vi "Dual_image_synced_p_read.vi"() -> ()   [LabVIEW 2013]
uses:
  <vilib>/DAQmx/write.llb/DAQmx Write (Analog DBL 1Chan 1Samp).vi
  <vilib>/DAQmx/create/channels.llb/DAQmx Create Channel (AO-Voltage-Basic).vi
  <vilib>/DAQmx/create/channels.llb/DAQmx Create Channel (CO-Pulse Generation-Frequency).vi
  <vilib>/DAQmx/configure/timing.llb/DAQmx Timing (Implicit).vi
  <vilib>/DAQmx/miscellaneous.llb/DAQmx Fill In Error Info.vi
  <vilib>/vision/driver/NI_Vision_Acquisition_Software.lvlib
  <resource>/objmgr/imaqdx.rc
  <resource>/objmgr/daqmx.rc
panel:
  in  "Pressure Frequency (Hz)":dbl=10.0 format="%#_13g"
  in  "im num 2":string
  in  "im time 2":string
  out "im num":string
  out "im time":string
  out "Pressure Reading":cluster{dbl[], dbl[]}(graph)
  in  "Pressure Offset":dbl
  out "Current Pressure (Psi)":dbl format="%#.4g"
  in  "Gain 2":dbl(slide)=575.0 min=350.0 max=1000.0 step=1.0 scale=350.0..1000.0
  in  "VR2":dbl(slide)=65.0 min=0.0 max=255.0 step=1.0 scale=0.0..255.0
  in  "VR1":dbl(slide)=60.0 min=0.0 max=255.0 step=1.0 scale=0.0..255.0
  in  "UB2":dbl(slide)=160.0 min=0.0 max=255.0 step=1.0 scale=0.0..255.0
  in  "UB1":dbl(slide)=165.0 min=0.0 max=255.0 step=1.0 scale=0.0..255.0
  in  "Shutter":dbl(slide)=4095.0 min=0.0 max=4095.0 step=1.0 scale=4.095..4095.0 scale format="%#.0f"
  in  "Brightness":dbl(slide)=100.0 min=0.0 max=255.0 step=1.0 scale=0.0..255.0
  in  "Gain":dbl(slide)=600.0 min=350.0 max=1000.0 step=1.0 scale=350.0..1000.0
  in  "Test Description":string="test"
  in  "Storage Directory":path=path "C:/Users/Regen/Desktop/Users/Ryan Gergely/3D_DIC"
  out "Image 2":T1(plugin-control)
  out "Buffer Number 2":u32
  out "Frame Rate 2":dbl
  in  "Camera Name 2":refnum<k21>="cam2" caption="IMAQdx Session"
  in  "Image Frequency (Hz)":dbl=2.0 format="%.1f"
  out "Actual Duty Cycle":dbl
  out "Actual Frequency":dbl
  in  "Stop":bool
  in  "Start Trigger Mode":bool
  out "Frame Rate 1":dbl
  out "Buffer Number 1":u32
  in  "Camera Name 1":refnum<k21>="cam1" caption="IMAQdx Session"
  out "Image":T1(plugin-control)
  # "Exposure Settings - Both Cameras"
  # "White Balance - Camera1"
  # "White Balance - Camera2"
  # "1) Set Test Description and Storage Directory"
  # "2) Select Cameras"
  # "3) Start VI"
  # "4) Set Frequency and Exposure and White Balance\n(Before Start Trigger)"
  # "5)"
  # "6) Stop When Done"
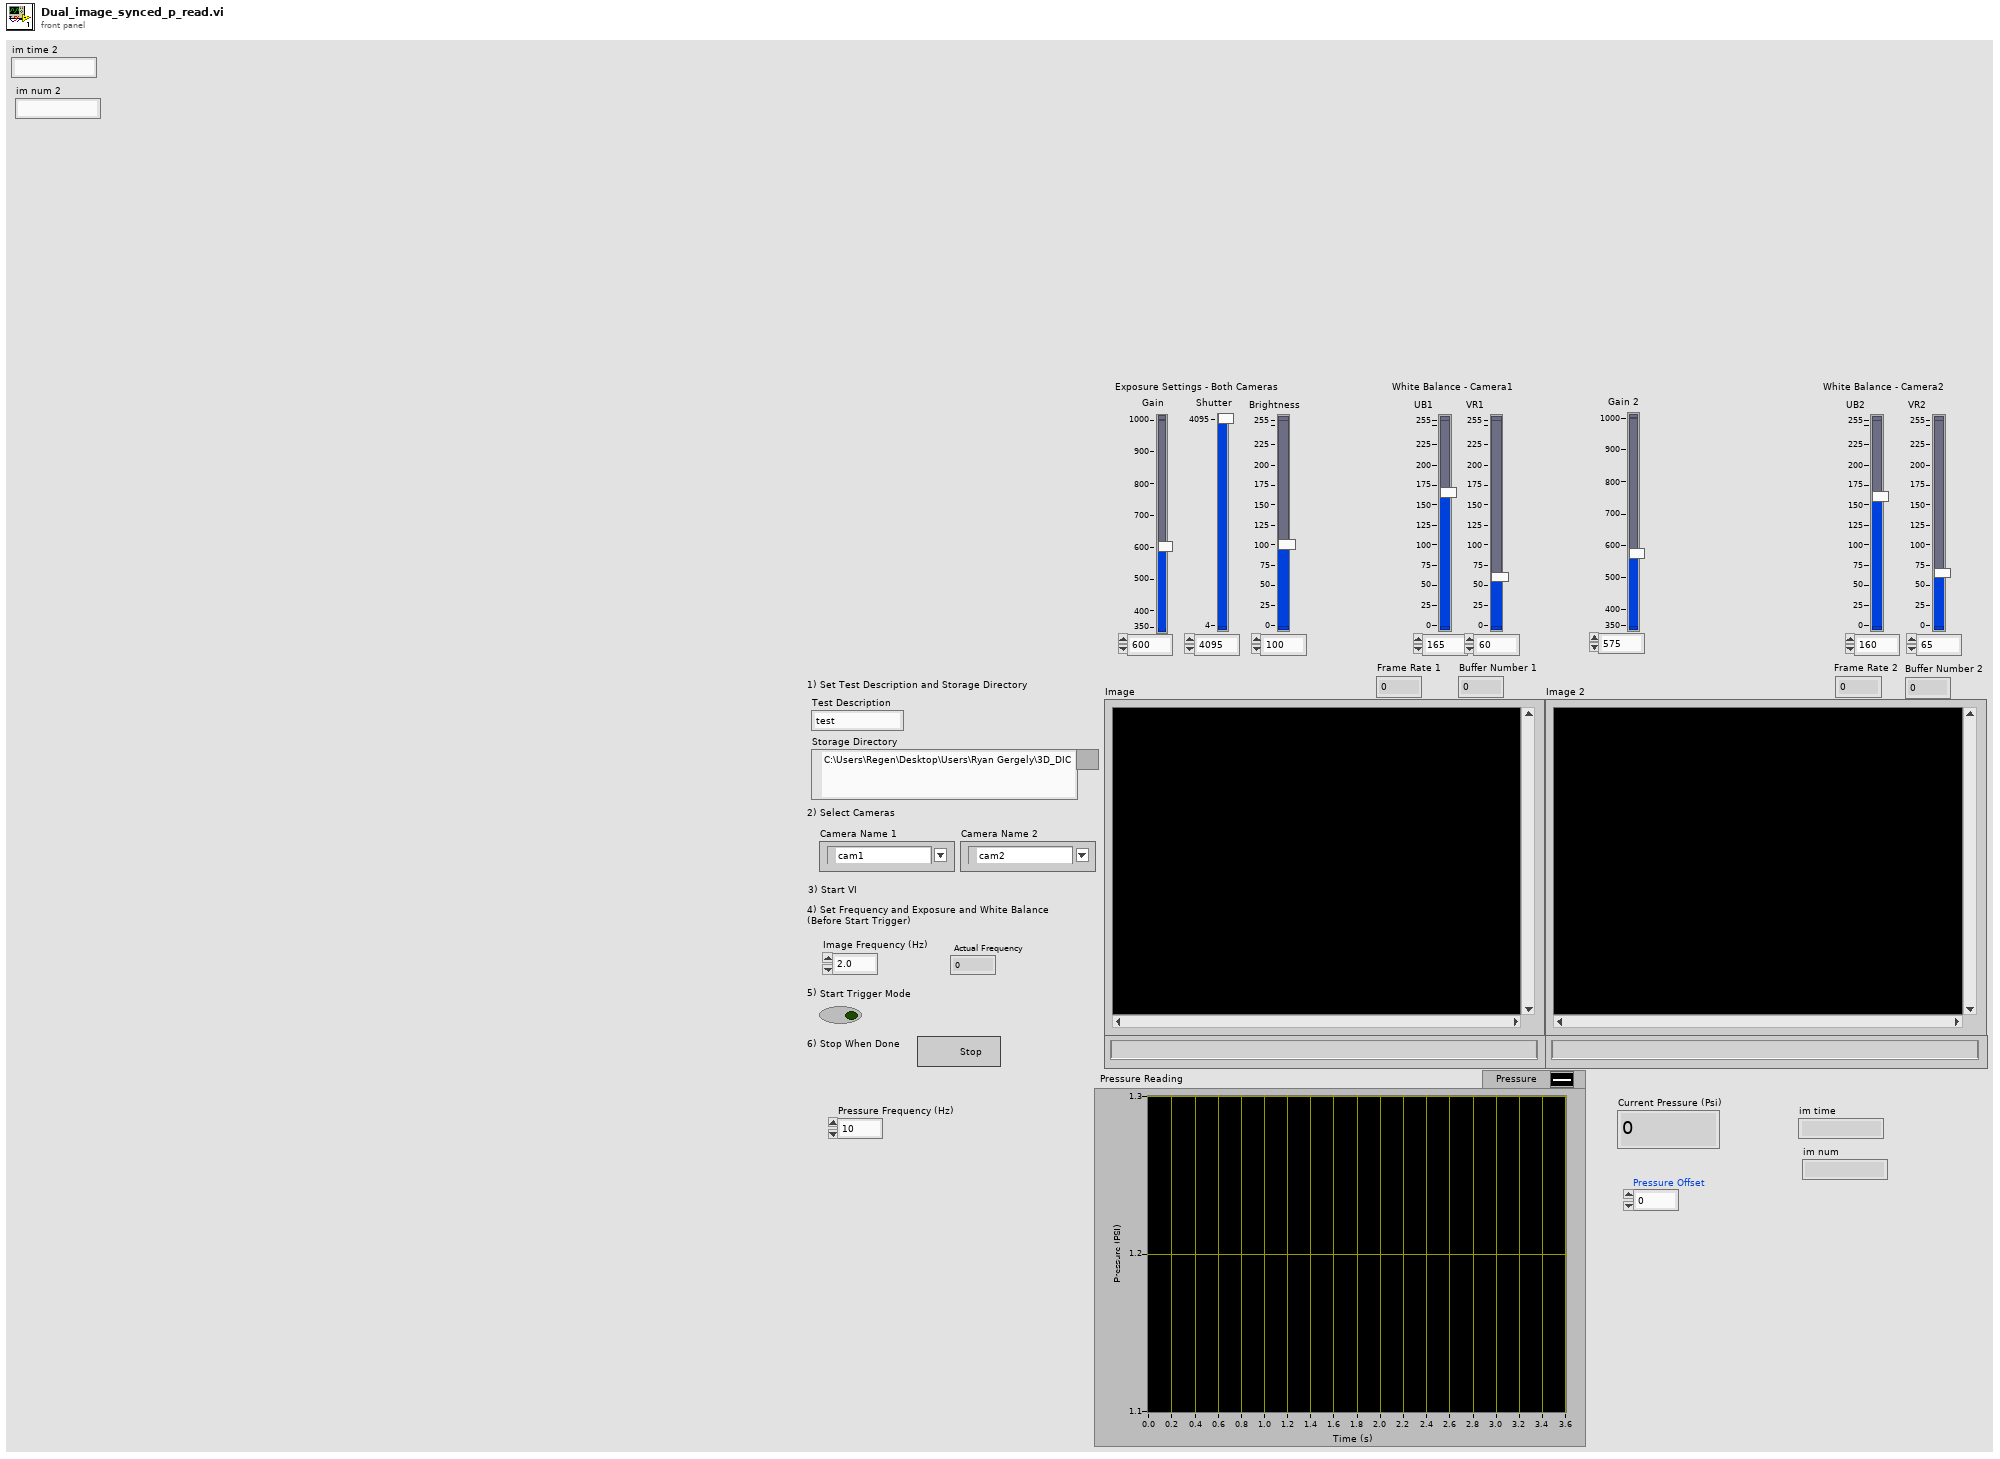
[diagram p1: front panel]
types:
  T1 = typedef "IMAQ Image.ctl" = refnum<image>
  T2 = enum16{"open", "open or create", "create or replace", "create", "open (read only)"}
  T3 = typedef "IMAQdx.ctl" = refnum<k21>
  T4 = cluster{"Trigger Mode":u32, "Trigger Activation":u32, "Timeout (ms)":u32}
  T5 = enum16{"open", "replace", "create", "open or create", "replace or create", "replace or create with confirmation"}
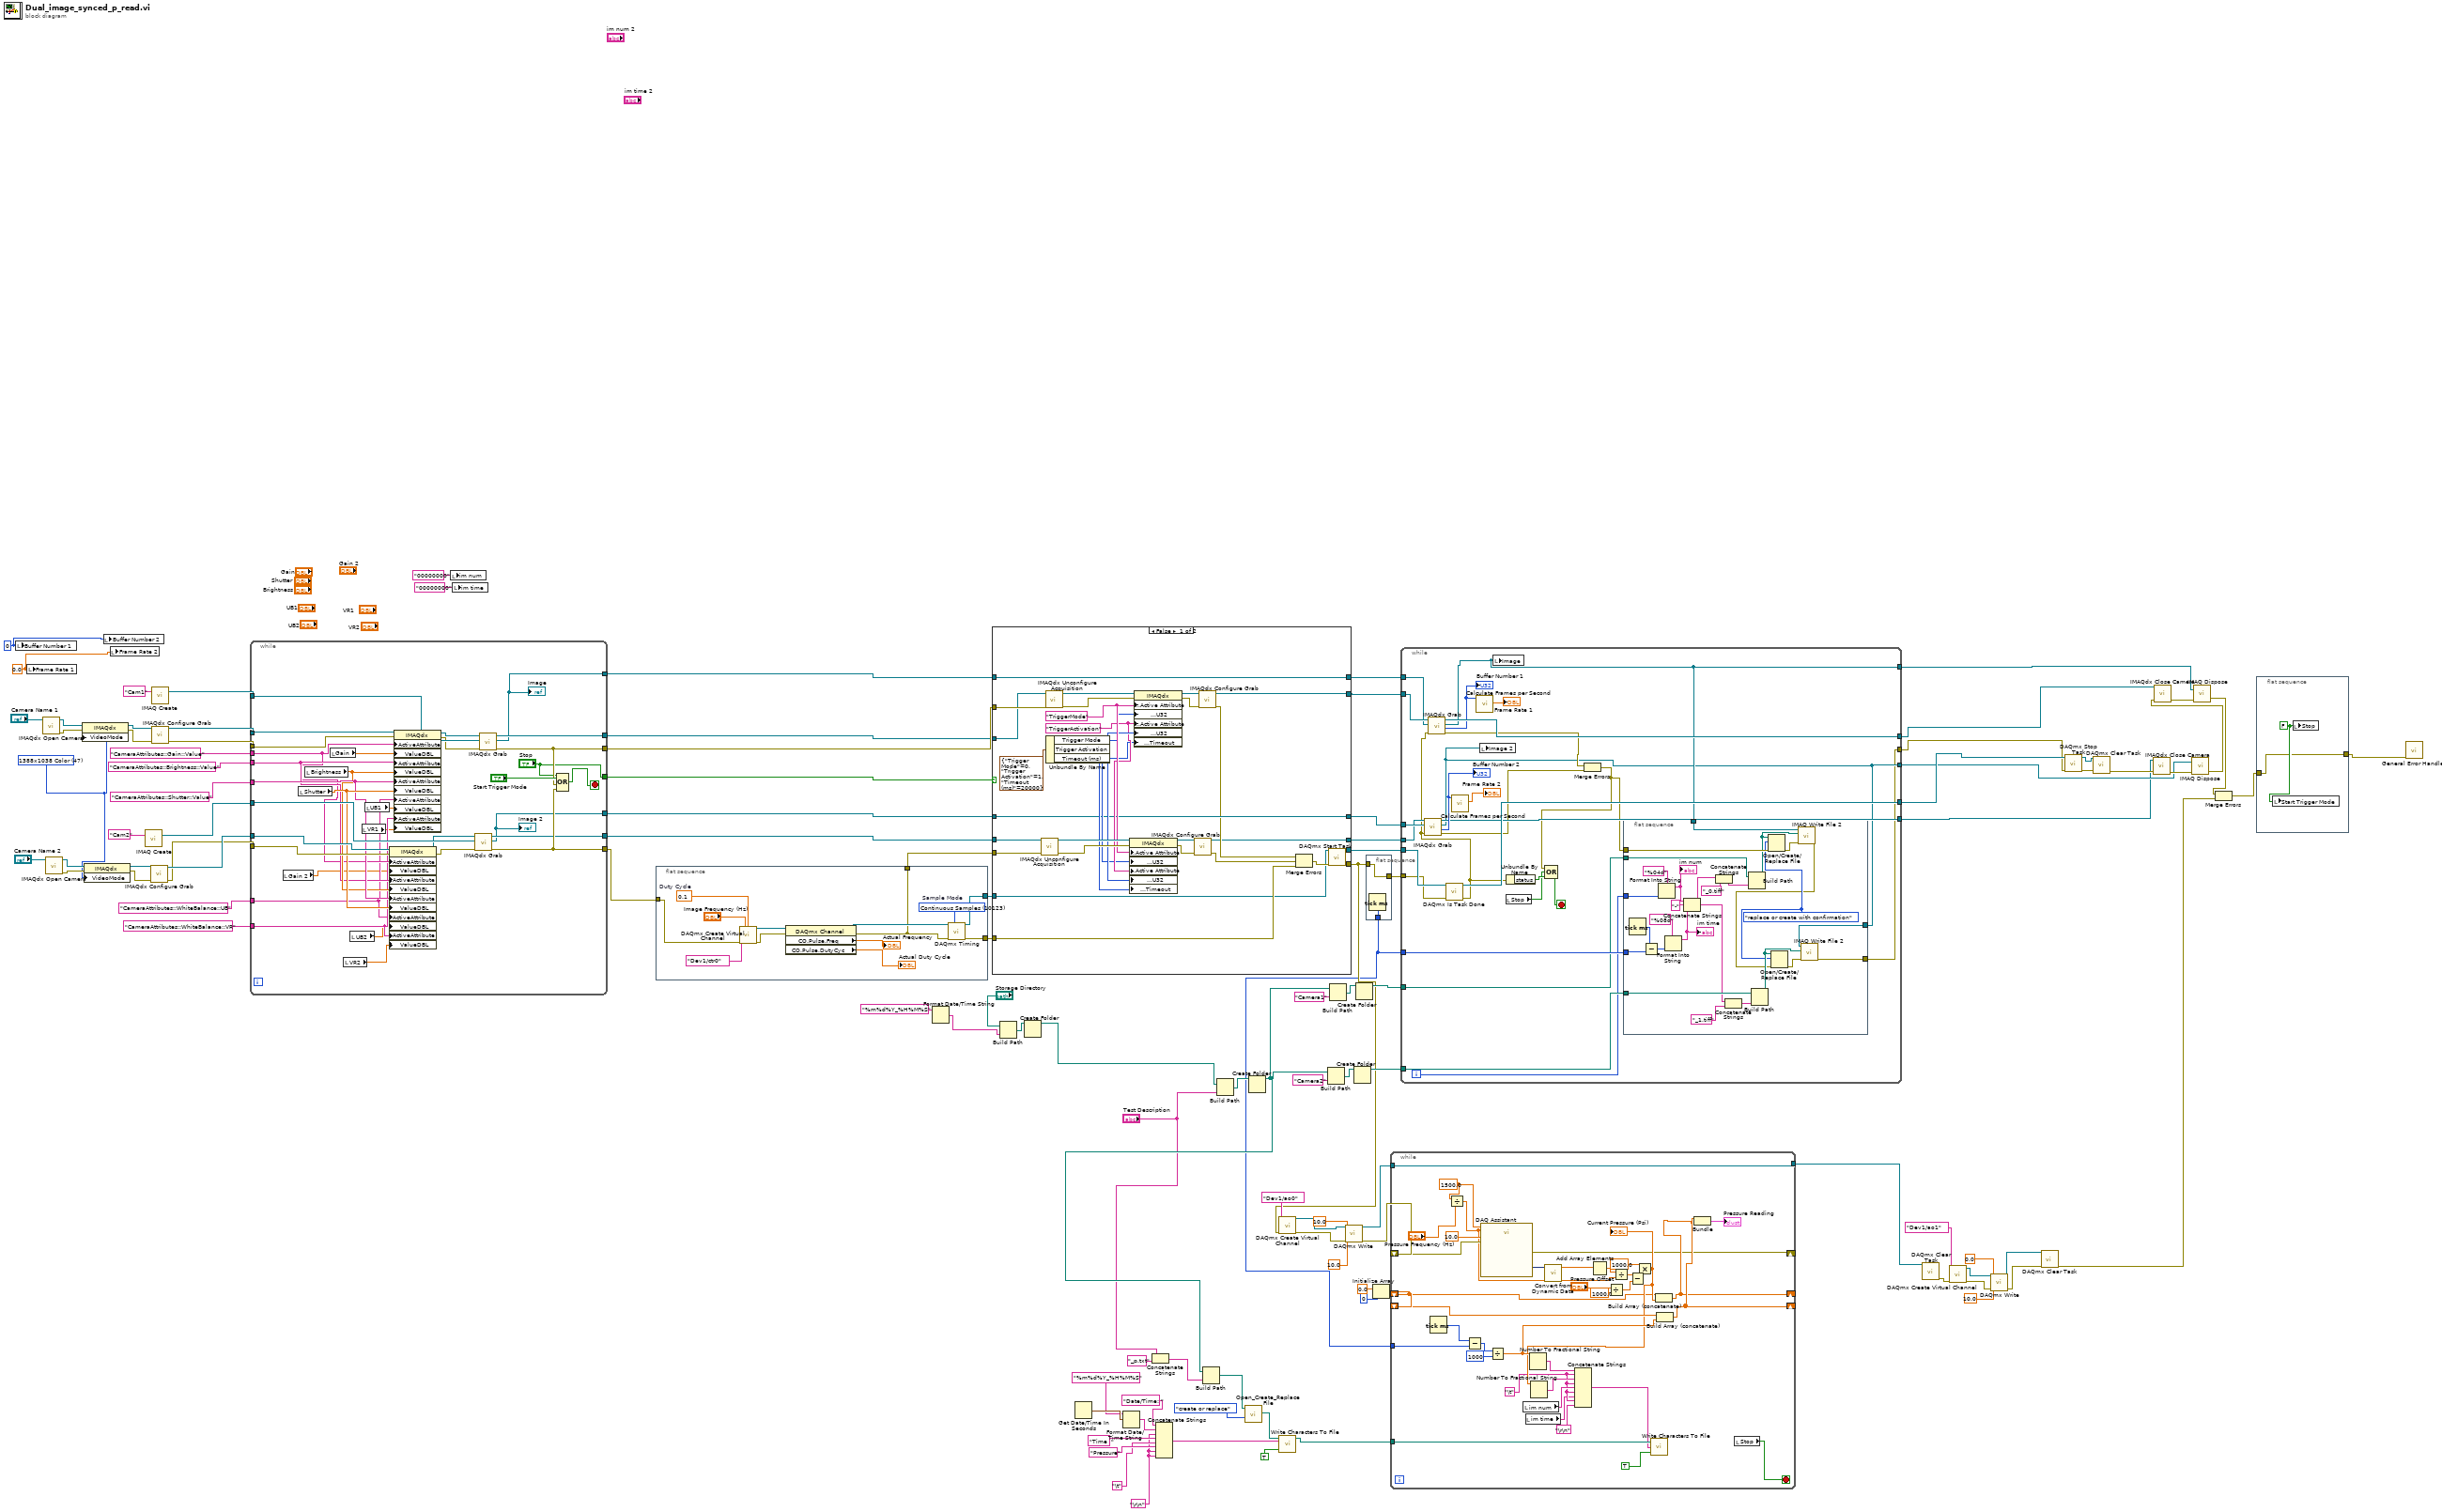
[diagram p0: block diagram]
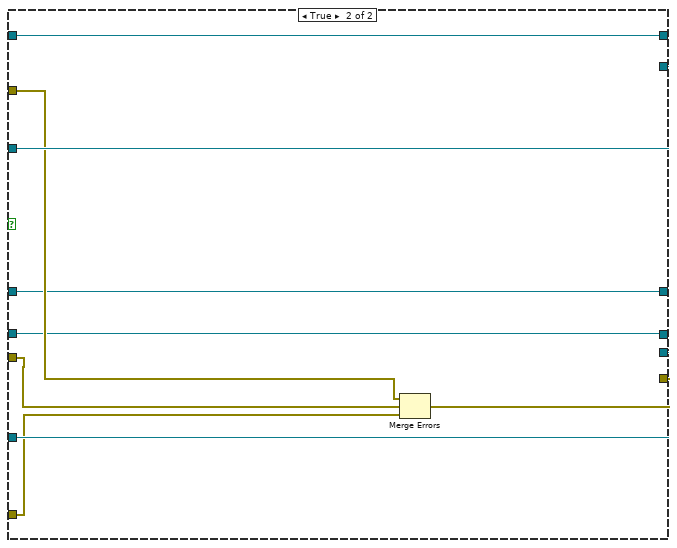
[diagram p2: hidden frame]
diagram:
  w34 = "\r\n"
  w57 = u32 47 items=["320x240 Color"=4, "640x480 Mono8"=9, "640x480 Mono16"=19, "640x480 Color"=14, "800x600 Mono8"=21, "800x600 Mono16"=27, "800x600 Color"=24, "1024x768 Mono8"=30, "1024x768 Mono16"=36, "1024x768 Color"=33, "1280x960 Mono8"=40, "1280x960 Mono16"=46, "1280x960 Color"=43, "1388x1038 Color"=47, "1388x1038 Mono"=48] ("Video Mode")
  w58 = 0.0 ("Frame Rate 1")
  w59 = u32 0 ("Buffer Number 1")
  n1 = local write "Buffer Number 1"(w59) -> ()
  n2 = local write "Frame Rate 1"(w58) -> ()
  n3 = call <vilib>:"IMAQdx Open Camera.vi"("Session In"="Camera Name 1") -> ("error out"=w65:errorcluster, "Session Out"=w67:T3)  [unwired: 2 in, 7 out]
  n4 = call <vilib>:"IMAQdx Open Camera.vi"("Session In"="Camera Name 2") -> ("error out"=w60:errorcluster, "Session Out"=w61:T3)  [unwired: 2 in, 7 out]
  n5 = property class="IMAQdx"(reference=w67, error in=w65, "VideoMode"=w57) -> (reference out=w66:T3, error out=w64:errorcluster)
  n6 = property class="IMAQdx"(reference=w61, error in=w60, "VideoMode"=w57) -> (reference out=w63:T3, error out=w62:errorcluster)
  n7 = local write "Buffer Number 2"(w59) -> ()
  n8 = local write "Frame Rate 2"(w58) -> ()
  n9 = call "IMAQ Create"("Image Name"="Cam2") -> ("New Image"=w54:T1)  [unwired: 3 in, 2 out]
  n10 = call <vilib>:"IMAQdx Configure Grab.vi"("error in"=w62, "Session In"=w63) -> ("error out"=w90:errorcluster, "Session Out"=w91:T3)  [unwired: 8 out]
  n11 = call "IMAQ Create"("Image Name"="Cam1") -> ("New Image"=w101:T1)  [unwired: 3 in, 2 out]
  n12 = call <vilib>:"IMAQdx Configure Grab.vi"("error in"=w64, "Session In"=w66) -> ("error out"=w99:errorcluster, "Session Out"=w100:T3)  [unwired: 8 out]
  n13 = while {
    tunnel: [w143] -> w108
    tunnel: w99 -> [w130]
    tunnel: w100 -> [w132]
    tunnel: [w139] -> w109
    tunnel: w101 -> [w134]
    tunnel: [w142] -> w96
    tunnel: ["Stop"] -> w97
    tunnel: w91 -> [w128]
    tunnel: w90 -> [w127]
    tunnel: [w137] -> w56
    tunnel: [w136] -> w89
    tunnel: [w135] -> w88
    tunnel: w54 -> [w133]
    tunnel: "CameraAttributes::Shutter::Value" ("ActiveAttribute") -> [w123]
    tunnel: "CameraAttributes::Brightness::Value" ("ActiveAttribute") -> [w121]
    tunnel: "CameraAttributes::Gain::Value" ("ActiveAttribute") -> [w119]
    tunnel: "CameraAttributes::WhiteBalance::UB" ("ActiveAttribute") -> [w116]
    tunnel: "CameraAttributes::WhiteBalance::VR" ("ActiveAttribute") -> [w117]
    stop <- w140 stop-if-true
    n14 = local read "Gain 2"() -> (w112:dbl)
    n15 = local read "Shutter"() -> (w124:dbl)
    n16 = local read "Brightness"() -> (w122:dbl)
    n17 = local read "Gain"() -> (w120:dbl)
    n18 = local read "VR2"() -> (w113:dbl)
    n19 = local read "UB2"() -> (w115:dbl)
    n20 = local read "VR1"() -> (w114:dbl)
    n21 = local read "UB1"() -> (w118:dbl)
    n22 = property class="IMAQdx"(reference=w128, error in=w127, "ActiveAttribute"=w119, "ValueDBL"=w112, "ActiveAttribute"=w121, "ValueDBL"=w122, "ActiveAttribute"=w123, "ValueDBL"=w124, "ActiveAttribute"=w116, "ValueDBL"=w115, "ActiveAttribute"=w117, "ValueDBL"=w113) -> (reference out=w125:T3, error out=w126:errorcluster)
    n23 = property class="IMAQdx"(reference=w132, error in=w130, "ActiveAttribute"=w119, "ValueDBL"=w120, "ActiveAttribute"=w121, "ValueDBL"=w122, "ActiveAttribute"=w123, "ValueDBL"=w124, "ActiveAttribute"=w116, "ValueDBL"=w118, "ActiveAttribute"=w117, "ValueDBL"=w114) -> (reference out=w131:T3, error out=w129:errorcluster)
    n24 = call <vilib>:"IMAQdx Grab.vi"("error in"=w126, "Image In"=w133, "Session In"=w125) -> ("error out"=w137:errorcluster, "Image Out"=w135:T1, "Session Out"=w136:T3)  [unwired: 1 in, 5 out]
    "Image 2" <- w135
    n25 = call <vilib>:"IMAQdx Grab.vi"("error in"=w129, "Image In"=w134, "Session In"=w131) -> ("error out"=w139:errorcluster, "Image Out"=w142:T1, "Session Out"=w143:T3)  [unwired: 1 in, 5 out]
    "Image" <- w142
    n26 = Compound Arithmetic op=OR("Stop", "Start Trigger Mode", w139, w137) -> (w140:bool)
  }
  n27 = local write "im num"("00000000" ("im num 2")) -> ()
  n28 = local write "im time"("00000000" ("im time 2")) -> ()
  n29 = flat-sequence {
    tunnel: [w147] -> w94
    tunnel: [w146] -> w87
    tunnel: w56 -> [w145]
    tunnel: [w144] -> w55
    frame #0 {
      w154 = 0.1  # Duty Cycle
      w148 = 10123 items=["Finite Samples"=10178, "Continuous Samples"=10123, "Hardware Timed Single Point"=12522]  # Sample Mode
      n30 = call-poly <vilib>:"DAQmx Create Virtual Channel.vi"("frequency"="Image Frequency (Hz)", "duty cycle"=w154, "counter"=tag "Dev1/ctr0" ("Counter"), "error in"=w145) -> ("task out"=w150:refnum<k21>, "error out"=w151:errorcluster)  [unwired: 10 in]
      n31 = property class="DAQmx Channel"(reference=w150, error in=w151) -> (reference out=w152:refnum<k21>, error out=w144:errorcluster, "CO.Pulse.Freq"=→"Actual Frequency":dbl, "CO.Pulse.DutyCyc"=→"Actual Duty Cycle":dbl)
      n32 = call-poly <vilib>:"DAQmx Timing.vi"("task/channels in"=w152, "sample mode"=w148, "error in"=w144) -> ("task out"=w147:refnum<k21>, "error out"=w146:errorcluster)  [unwired: 11 in]
    }
  }
  n33 = Format Date/Time String(time format string (%c)="%m%d%Y_%H%M%S") -> (date/time string=w76:string)  [unwired: 2 in]
  n34 = case shown="False" w97 {
    tunnel: w109 -> [w185 w191]
    tunnel: w108 -> [w184 w194]
    tunnel: [w183 w194] -> w107
    tunnel: [w164 w190] -> w9
    tunnel: [w165 w192] -> w105
    tunnel: w96 -> [w177 w193]
    tunnel: [w177 w193] -> w95
    tunnel: w94 -> [w157 w192]
    tunnel: w55 -> [w168 w189]
    tunnel: w89 -> [w167 w186]
    tunnel: w88 -> [w166 w187]
    tunnel: [w166 w187] -> w86
    tunnel: w87 -> [w160 w188]
    tunnel: [w158 w186] -> w85
    frame False {
      w171 = "TriggerActivation" ("ActiveAttribute")
      w173 = "TriggerMode" ("ActiveAttribute")
      n35 = call <vilib>:"IMAQdx Unconfigure Acquisition.vi"("error in"=w168, "Session In"=w167) -> ("error out"=w175:errorcluster, "Session Out"=w174:T3)  [unwired: 8 out]
      n36 = call <vilib>:"IMAQdx Unconfigure Acquisition.vi"("error in"=w185, "Session In"=w184) -> ("error out"=w180:errorcluster, "Session Out"=w179:T3)  [unwired: 8 out]
      n37 = Unbundle By Name(T4 {"Trigger Mode"=0, "Trigger Activation"=1, "Timeout (ms)"=20000} ("Trigger Parameters")) -> ("Trigger Mode"=w169:u32, "Trigger Activation"=w172:u32, "Timeout (ms)"=w170:u32)
      n38 = property class="IMAQdx"(reference=w174, error in=w175, "Camera Attributes:Active Attribute"=w173, "Camera Attributes:Value:U32"=w169, "Camera Attributes:Active Attribute"=w171, "Camera Attributes:Value:U32"=w172, "Acquisition Attributes:Timeout"=w170) -> (reference out=w176:T3, error out=w163:errorcluster)
      n39 = property class="IMAQdx"(reference=w179, error in=w180, "Camera Attributes:Active Attribute"=w173, "Camera Attributes:Value:U32"=w169, "Camera Attributes:Active Attribute"=w171, "Camera Attributes:Value:U32"=w172, "Acquisition Attributes:Timeout"=w170) -> (reference out=w181:T3, error out=w182:errorcluster)
      n40 = call <vilib>:"IMAQdx Configure Grab.vi"("error in"=w163, "Session In"=w176) -> ("error out"=w161:errorcluster, "Session Out"=w158:T3)  [unwired: 8 out]
      n41 = call <vilib>:"IMAQdx Configure Grab.vi"("error in"=w182, "Session In"=w181) -> ("error out"=w159:errorcluster, "Session Out"=w183:T3)  [unwired: 8 out]
      n42 = Merge Errors(w159, w161, w160) -> (w162:errorcluster)
      n43 = call <vilib>:"DAQmx Start Task.vi"("task/channels in"=w157, "error in"=w162) -> ("task out"=w165:refnum<k21>, "error out"=w164:errorcluster)  [unwired: 12 in]
    }
    frame True {
      n44 = Merge Errors(w191, w189, w188) -> (w190:errorcluster)
    }
  }
  n45 = Build Path(base path="Storage Directory", name or relative path=w76) -> (appended path=w78:path)
  n46 = Create Folder(path (use dialog)=w78) -> (created path=w21:path)  [unwired: 2 in, 2 out]
  n47 = Get Date/Time In Seconds() -> (seconds since 1Jan1904=w33:timestamp)
  n48 = Format Date/Time String(time format string (%c)="%m%d%Y_%H%M%S", seconds (now)=w33) -> (date/time string=w41:string)  [unwired: 1 in]
  n49 = Concatenate Strings("Test Description", "_p.txt" ("string")) -> (w46:string)
  n50 = Concatenate Strings("Date/Time: ", w41, w34, "Time  ", "\t", "Pressure" ("string"), w34, w34) -> (w42:string)
  n51 = Build Path(base path=w21, name or relative path="Test Description") -> (appended path=w74:path)
  n52 = Create Folder(path (use dialog)=w74) -> (created path=w20:path)  [unwired: 2 in, 2 out]
  n53 = Build Path(base path=w20, name or relative path=w46) -> (appended path=w38:path)
  n54 = call <vilib>:"Open_Create_Replace File.vi"("function (open:0)"=T2."create or replace", "file path"=w38) -> ("new file path"=w44:path)  [unwired: 6 in, 3 out]
  n55 = call-poly <vilib>:"DAQmx Create Virtual Channel.vi"("physical channels"=tag "Dev1/ao0", "error in"=w9) -> ("task out"=w24:refnum<k21>, "error out"=w28:errorcluster)  [unwired: 12 in]
  n56 = call <vilib>:"Write Characters To File.vi"("append to file? (new file:F)"=TRUE, "character string"=w42, "file path (dialog if empty)"=w44) -> ("new file path (Not A Path if cancelled)"=w37:path)  [unwired: 2 in]
  n57 = Build Path(base path=w20, name or relative path="Camera2") -> (appended path=w69:path)
  n58 = Build Path(base path=w20, name or relative path="Camera1") -> (appended path=w72:path)
  n59 = call-poly <vilib>:"DAQmx Write.vi"("task/channels in"=w24, "data"=10.0, "timeout"=10.0, "error in"=w28) -> ("task out"=w22:refnum<k21>, "error out"=w23:errorcluster)  [unwired: 9 in, 1 out]
  n60 = Create Folder(path (use dialog)=w69) -> (created path=w68:path)  [unwired: 2 in, 2 out]
  n61 = Create Folder(path (use dialog)=w72) -> (created path=w71:path)  [unwired: 2 in, 2 out]
  n62 = flat-sequence {
    tunnel: w9 -> [w196]
    tunnel: [w196] -> w48
    tunnel: [w195] -> w8
    frame #0 {
      n63 = Tick Count (ms)() -> (millisecond timer value=w195:u32)
    }
  }
  n64 = Initialize Array(0.0 ("element"), 0 ("dimension size")) -> (w30:dbl[])
  n65 = while {
    tunnel: w37 -> [w233]
    tunnel: w8 -> [w230]
    shift-right: [w208] -> _
    shift-left: w23 -> [w223]
    shift-right: [w215] -> _
    shift-left: w30 -> [w209]
    shift-right: [w216] -> _
    shift-left: w30 -> [w218]
    tunnel: w22 -> [w214]
    tunnel: [w214] -> w11
    stop <- w198 stop-if-true
    w204 = 1500.0 ("rate")
    w201 = "\t"
    n66 = Tick Count (ms)() -> (millisecond timer value=w231:u32)
    n67 = Divide(x=w204, y="Pressure Frequency (Hz)") -> (x/y=w203:dbl)
    n68 = Subtract(x=w231, y=w230) -> (x-y=w229:u32)
    n69 = call "DAQ Assistant"("rate"=w204, "number of samples"=w203, "timeout (s)"=10.0, "error in"=w223) -> ("data"=w224:dynamicdata, "error out"=w208:errorcluster)  [unwired: 13 in, 1 out]
    n70 = Divide(x=w229, y=u32 1000) -> (x/y=w219:dbl)
    n71 = local read "im num"() -> (w202:string)
    n72 = local read "im time"() -> (w200:string)
    n73 = Number To Fractional String(number=w219) -> (F-format string=w227:string)  [unwired: 3 in]
    n74 = call "Convert from Dynamic Data"("Dynamic Data Type"=w224) -> ("Array"=w221:dbl[])  [unwired: 3 in]
    n75 = Add Array Elements(numeric array=w221) -> (sum=w220:dbl)
    n76 = Divide(x="Pressure Offset", y=1000.0) -> (x/y=w205:dbl)
    n77 = Divide(x=w220, y=w203) -> (x/y=w213:dbl)
    n78 = Subtract(x=w213, y=w205) -> (x-y=w211:dbl)
    n79 = Multiply(x=w211, y=1000.0) -> (x*y=w210:dbl)
    "Current Pressure (Psi)" <- w210
    n80 = Number To Fractional String(number=w210) -> (F-format string=w226:string)  [unwired: 3 in]
    n81 = Concatenate Strings(w227, w201, w226, w201, w202, w201, w200, w201, "\r\n") -> (w225:string)
    n82 = call <vilib>:"Write Characters To File.vi"("append to file? (new file:F)"=TRUE, "character string"=w225, "file path (dialog if empty)"=w233) -> ()  [unwired: 2 in, 1 out]
    n83 = Build Array (concatenate)(w209, w210) -> (w215:dbl[])
    n84 = Build Array (concatenate)(w218, w219) -> (w216:dbl[])
    n85 = Bundle(w216, w215) -> (→"Pressure Reading":cluster{dbl[], dbl[]})  [unwired: 1 in]
    n86 = local read "Stop"() -> (w198:bool)
  }
  n87 = while {
    tunnel: [w260] -> w103
    tunnel: [w238] -> w3
    tunnel: w107 -> [w257]
    tunnel: w95 -> [w256]
    tunnel: [w253] -> w102
    tunnel: w105 -> [w252]
    tunnel: w86 -> [w249]
    tunnel: w85 -> [w248]
    tunnel: w48 -> [w245]
    tunnel: [w242] -> w79
    tunnel: [w241] -> w81
    tunnel: [w244] -> w80
    tunnel: w71 -> [w235]
    tunnel: w68 -> [w243]
    tunnel: w8 -> [w237]
    i -> [w234]
    stop <- w254 stop-if-true
    n88 = call <vilib>:"DAQmx Is Task Done.vi"("task/channels in"=w252, "error in"=w245) -> ("task out"=w253:refnum<k21>, "error out"=w239:errorcluster)  [unwired: 11 in, 1 out]
    n89 = call <vilib>:"IMAQdx Grab.vi"("error in"=w239, "Image In"=w249, "Session In"=w248) -> ("error out"=w240:errorcluster, "Buffer Number Out"=w247:u32, "Image Out"=w241:T1, "Session Out"=w244:T3)  [unwired: 1 in, 4 out]
    "Buffer Number 2" <- w247
    n90 = call <vilib>:"IMAQdx Grab.vi"("error in"=w239, "Image In"=w256, "Session In"=w257) -> ("error out"=w246:errorcluster, "Buffer Number Out"=w258:u32, "Image Out"=w242:T1, "Session Out"=w260:T3)  [unwired: 1 in, 4 out]
    "Buffer Number 1" <- w258
    n91 = call <vilib>:"Calculate Frames per Second.vi"("Buffer Number"=w247) -> ("Processed Frames/s"=→"Frame Rate 2":dbl)  [unwired: 8 in, 2 out]
    n92 = call <vilib>:"Calculate Frames per Second.vi"("Buffer Number"=w258) -> ("Processed Frames/s"=→"Frame Rate 1":dbl)  [unwired: 8 in, 2 out]
    n93 = local write "Image 2"(w241) -> ()
    n94 = local write "Image"(w242) -> ()
    n95 = Unbundle By Name(w239) -> ("status"=w255:bool)
    n96 = local read "Stop"() -> (w251:bool)
    n97 = Merge Errors(w246, w240) -> (w236:errorcluster)
    n98 = Compound Arithmetic op=OR(w236, w251, w255) -> (w254:bool)
    n99 = flat-sequence {
      tunnel: w235 -> [w286]
      tunnel: w243 -> [w285]
      tunnel: w242 -> [w284]
      tunnel: w241 -> [w283]
      tunnel: w236 -> [w282]
      tunnel: [w281] -> w238
      tunnel: w237 -> [w274]
      tunnel: w234 -> [w266]
      frame #0 {
        w278 = T5."replace or create with confirmation" ("operation (0:open)")
        n100 = Tick Count (ms)() -> (millisecond timer value=w273:u32)
        n101 = Subtract(x=w273, y=w274) -> (x-y=w269:u32)
        n102 = Format Into String(format string="%04d", w266) -> (resulting string=w264:string)  [unwired: 2 in, 1 out]
        "im num" <- w264
        n103 = Format Into String(format string="%08d", w269) -> (resulting string=w268:string)  [unwired: 2 in, 1 out]
        "im time" <- w268
        n104 = Concatenate Strings(w264, "-" ("string"), w268) -> (w261:string)
        n105 = Concatenate Strings(w261, "_0.tiff") -> (w271:string)
        n106 = Concatenate Strings(w261, "_1.tiff") -> (w272:string)
        n107 = Build Path(base path=w286, name or relative path=w271) -> (appended path=w280:path)
        n108 = Build Path(base path=w285, name or relative path=w272) -> (appended path=w279:path)
        n109 = Open/Create/Replace File(file path (use dialog)=w280, error in=w282, operation (0:open)=w278) -> (error out=w277:errorcluster)  [unwired: 3 in, 2 out]
        n110 = call-poly "IMAQ Write File 2"("error in (no error)"=w277, "File Path"=w280, "Image"=w284) -> ("error out"=w275:errorcluster)  [unwired: 7 in, 1 out]
        n111 = Open/Create/Replace File(file path (use dialog)=w279, error in=w275, operation (0:open)=w278) -> (error out=w276:errorcluster)  [unwired: 3 in, 2 out]
        n112 = call-poly "IMAQ Write File 2"("error in (no error)"=w276, "File Path"=w279, "Image"=w283) -> ("error out"=w281:errorcluster)  [unwired: 7 in, 1 out]
      }
    }
  }
  n113 = call <vilib>:"DAQmx Clear Task.vi"("task in"=w11) -> ("error out"=w18:errorcluster)  [unwired: 14 in]
  n114 = call-poly <vilib>:"DAQmx Create Virtual Channel.vi"("physical channels"=tag "Dev1/ao1", "error in"=w18) -> ("task out"=w13:refnum<k21>, "error out"=w19:errorcluster)  [unwired: 12 in]
  n115 = call-poly <vilib>:"DAQmx Write.vi"("task/channels in"=w13, "data"=0.0, "timeout"=10.0, "error in"=w19) -> ("task out"=w12:refnum<k21>, "error out"=w17:errorcluster)  [unwired: 9 in, 1 out]
  n116 = call <vilib>:"DAQmx Clear Task.vi"("task in"=w12, "error in"=w17) -> ("error out"=w6:errorcluster)  [unwired: 13 in]
  n117 = call <vilib>:"DAQmx Stop Task.vi"("task/channels in"=w102, "error in"=w3) -> ("task out"=w104:refnum<k21>, "error out"=w106:errorcluster)  [unwired: 12 in]
  n118 = call <vilib>:"DAQmx Clear Task.vi"("task in"=w104, "error in"=w106) -> ("error out"=w82:errorcluster)  [unwired: 13 in]
  n119 = call <vilib>:"IMAQdx Close Camera.vi"("error in"=w82, "Session In"=w80) -> ("error out"=w84:errorcluster)  [unwired: 9 out]
  n120 = call "IMAQ Dispose"("Image"=w81, "error in (no error)"=w84) -> ("error out"=w83:errorcluster)  [unwired: 4 in]
  n121 = call <vilib>:"IMAQdx Close Camera.vi"("error in"=w83, "Session In"=w103) -> ("error out"=w111:errorcluster)  [unwired: 9 out]
  n122 = call "IMAQ Dispose"("Image"=w79, "error in (no error)"=w111) -> ("error out"=w7:errorcluster)  [unwired: 4 in]
  n123 = Merge Errors(w7, w6) -> (w2:errorcluster)
  n124 = flat-sequence {
    tunnel: w2 -> [w287]
    tunnel: [w287] -> w1
    frame #0 {
      w288 = FALSE ("Stop")
      n125 = local write "Start Trigger Mode"(w288) -> ()
      n126 = local write "Stop"(w288) -> ()
    }
  }
  n127 = call <vilib>:"General Error Handler.vi"("error in (no error)"=w1) -> ()  [unwired: 1 in, 14 out]
